vi "Modbus Create.vi"(8 "error in (no error)":errorcluster) -> (0 "error out":errorcluster)   [LabVIEW 2011]
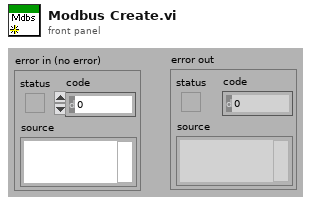
[diagram p1: front panel]
types:
  T1 = enum32{"Bad", "Idle", "Run top level", "Running"}
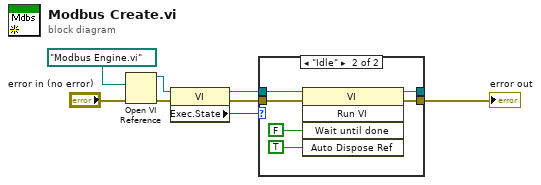
[diagram p0: block diagram]
diagram:
  n1 = Open VI Reference(vi path=path "Modbus Engine.vi", error in (no error)="error in (no error)") -> (vi reference=w6:refnum<vi>, error out=w5:errorcluster)  [unwired: 4 out]
  n2 = property class="VI"(reference=w6, error in=w5) -> (reference out=w3:refnum<vi>, error out=w2:errorcluster, "Exec.State"=w4:T1)
  n3 = case shown="\"Idle\"" w4 {
    tunnel: w3 -> [w10 w16]
    tunnel: [w10 w14] -> _
    tunnel: [w9 w13] -> w1
    tunnel: w2 -> [w9 w15]
    frame "Bad", Default {
    }
    frame "Idle" {
      n4 = invoke class="VI" method="Run VI"(reference=w16, error in=w15, "Wait until done"=FALSE ("Wait Until Done"), "Auto Dispose Ref"=TRUE ("Auto Dispose Reference")) -> (reference out=w14:refnum<vi>, error out=w13:errorcluster)  [unwired: 1 in, 3 out]
    }
  }
  "error out" <- w1
